vi "Setting Window.vi"() -> ()   [LabVIEW 2015]
panel:
  in  "Array":T1(array[cluster])
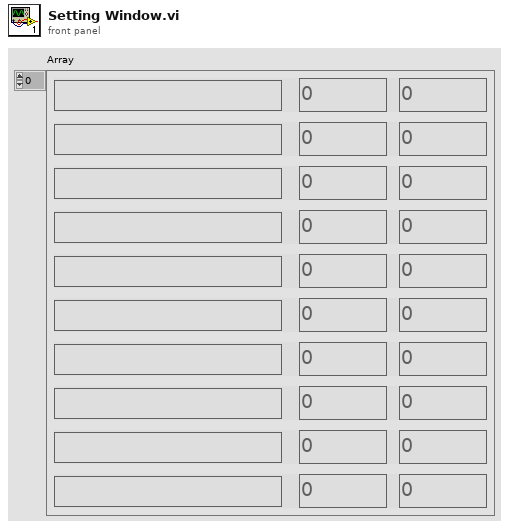
[diagram p1: front panel]
types:
  T1 = cluster{"Min Value":dbl, "sensor Nmae":string, "Max Value":dbl}[]
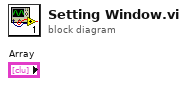
[diagram p0: block diagram]
diagram:
